vi "reached_setpoint.vi"(8 "error in":errorcluster, 10 "Setpoint value":dbl, 11 "Coarse Approach in":refnum<class "Coarse Approach.lvclass">) -> (0 "error out":errorcluster, 1 "Current value":dbl, 2 "Reached setpoint?":bool, 3 "Coarse Approach out":refnum<class "Coarse Approach.lvclass">, 4 "In Range?":bool)   [LabVIEW 2020, in "Coarse Approach.lvclass"]
uses:
  Coarse Approach.lvclass
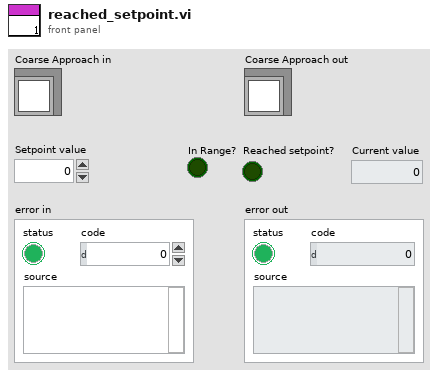
[diagram p1: front panel]
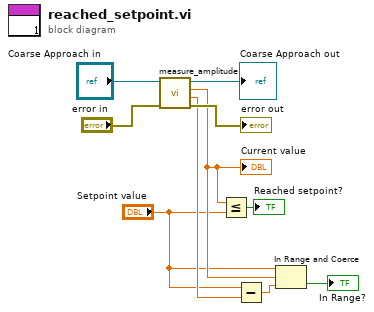
[diagram p0: block diagram]
diagram:
  n1 = call "measure_amplitude.vi"("error in"="error in", "Coarse Approach in"="Coarse Approach in") -> ("error out"=→"error out":errorcluster, "Amplitude stdev"=w4:dbl, "Amplitude mean"=w3:dbl, "Coarse Approach out"=→"Coarse Approach out":refnum<class "Coarse Approach.lvclass">)  [unwired: 6 in]
  "Current value" <- w3
  n2 = Less Or Equal?(x=w3, y="Setpoint value") -> (x <= y?=→"Reached setpoint?":bool)
  n3 = Subtract(x="Setpoint value", y=w4) -> (x-y=w5:dbl)
  n4 = In Range and Coerce(upper limit="Setpoint value", x=w3, lower limit=w5) -> (In Range?=→"In Range?":bool)  [unwired: 1 out]
